vi "Populate List Items.vi"(1 "List":string) -> (0 "Items":T1[](array[typedef]))   [LabVIEW 2020, in "AoC 2022.lvlib"]
uses:
  AoC 2022.lvlib
  Item.ctl
  Item Type.ctl
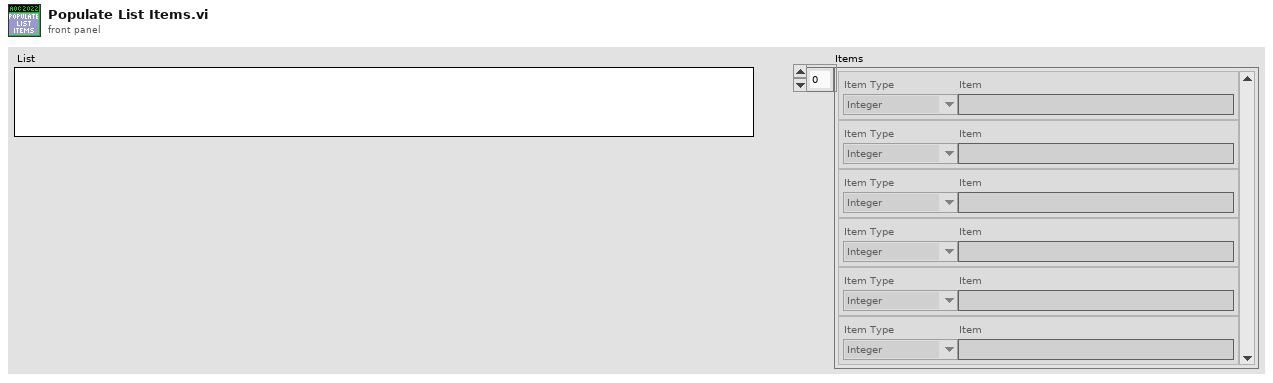
[diagram p1: front panel]
types:
  T1 = typedef "AoC 2022.lvlib/Item.ctl" = cluster{"Item Type":T2, "Item":string}
  T2 = typedef "AoC 2022.lvlib/Item Type.ctl" = enum16{"Integer", "List"}
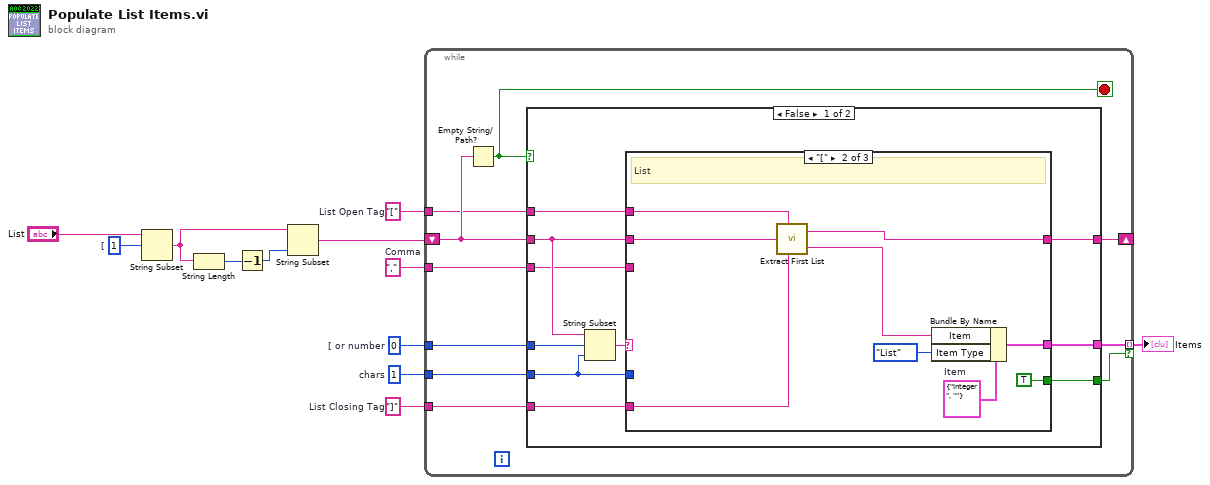
[diagram p0: block diagram]
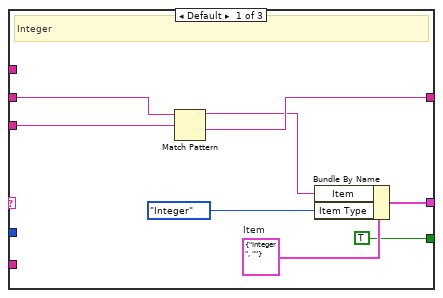
[diagram p2: hidden frame]
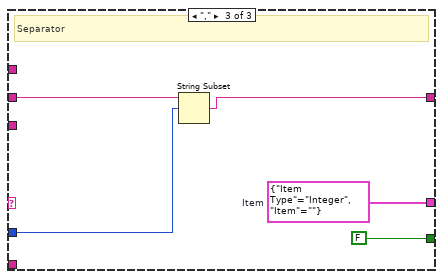
[diagram p3: hidden frame]
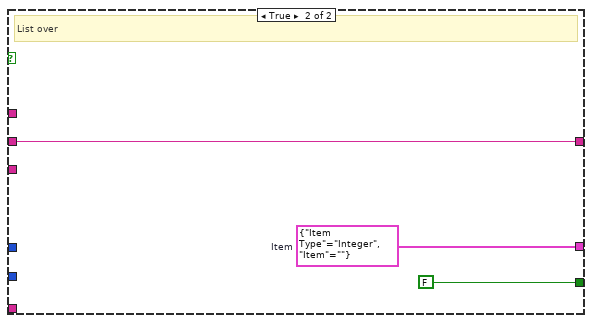
[diagram p4: hidden frame]
diagram:
  w1 = "["  # List Open Tag
  w2 = "]"  # List Closing Tag
  w4 = 1  # chars
  w8 = 0  # [ or number
  w6 = ","  # Comma
  w10 = 1  # [
  n1 = String Subset(string="List", offset (0)=w10) -> (substring=w11:string)  [unwired: 1 in]
  n2 = String Length(string=w11) -> (length=w12:i32)
  n3 = Decrement(x=w12) -> (x-1=w3:i32)
  n4 = String Subset(string=w11, length (rest)=w3) -> (substring=w7:string)  [unwired: 1 in]
  n5 = while {
    tunnel: w8 -> [w22]
    tunnel: w6 -> [w21]
    shift-right: [w20] -> _
    shift-left: w7 -> [w18]
    tunnel: [w19] -> w5 mode=indexing if=w16
    tunnel: w4 -> [w15]
    tunnel: w2 -> [w14]
    tunnel: w1 -> [w13]
    stop <- w17 stop-if-true
    n6 = Empty String/Path?(string/path=w18) -> (empty?=w17:bool)
    n7 = case shown="False" w17 {
      tunnel: w22 -> [w32 _]
      tunnel: w18 -> [w30 w55]
      tunnel: w21 -> [w29 _]
      tunnel: [w28 w55] -> w20
      tunnel: [w27 w57] -> w19
      tunnel: [w26 FALSE] -> w16
      tunnel: w15 -> [w25 _]
      tunnel: w14 -> [w24 _]
      tunnel: w13 -> [w23 _]
      frame False {
        n8 = String Subset(string=w30, offset (0)=w32, length (rest)=w25) -> (substring=w31:string)
        n9 = case shown="\"[\"" w31 {
          tunnel: w30 -> [w40 w43 w52]
          tunnel: w29 -> [w39 _ _]
          tunnel: [w38 w44 w50] -> w28
          tunnel: [w34 w47 w53] -> w27
          tunnel: [TRUE TRUE FALSE] -> w26
          tunnel: w25 -> [_ _ w51]
          tunnel: w24 -> [_ w42 _]
          tunnel: w23 -> [_ w41 _]
          frame Default {
            w37 = T1 {"Item Type"=enum."Integer", "Item"=""}  # Item
            # "Integer"
            n10 = Match Pattern(string=w40, regular expression=w39) -> (before substring=w35:string, after substring=w38:string)  [unwired: 1 in, 2 out]
            n11 = Bundle By Name(cluster=w37, "Item"=w35, "Item Type"=Item_Type."Integer") -> (w34:T1)
          }
          frame "[" {
            w49 = T1 {"Item Type"=enum."Integer", "Item"=""}  # Item
            # "List"
            n12 = call "Extract First List.vi"("List Open Tag"=w41, "String"=w43, "List Closing Tag"=w42) -> ("Remaining String"=w44:string, "First List"=w46:string)  [unwired: 2 in]
            n13 = Bundle By Name(cluster=w49, "Item"=w46, "Item Type"=Item_Type."List") -> (w47:T1)
          }
          frame "," {
            w53 = T1 {"Item Type"=enum."Integer", "Item"=""}  # Item
            # "Separator"
            n14 = String Subset(string=w52, offset (0)=w51) -> (substring=w50:string)  [unwired: 1 in]
          }
        }
      }
      frame True {
        w57 = T1 {"Item Type"=enum."Integer", "Item"=""}  # Item
        # "List over"
      }
    }
  }
  "Items" <- w5
